vi "LcError_SetError.vi"(1 "status":bool=TRUE, 2 "code (5000)":i32=5000, 3 "source":string, 5 "error in (no error)":errorcluster, 6 "UserDefinedCodes(+5000)":variant, 7 "Error SubVI Level(1)":i32=1, 8 "StartErrorCode(5000)":i32=5000) -> (19 "error out":errorcluster)   [LabVIEW 2019]
doc: "You can use this VI to generate errors.\nThe path to the calling Vi will be added in the source.\nIf you wrap this VI inside another SetError VI (E.g. MyApplication_SetError), you can change set the <B>Error SubVI Level(1)</B> to 2"
panel:
  # "If you wrap this VI inside another SetError VI (E.g. MyApplication_SetError), you can change set the <B>Error SubVI Level(1)</B> to 2"
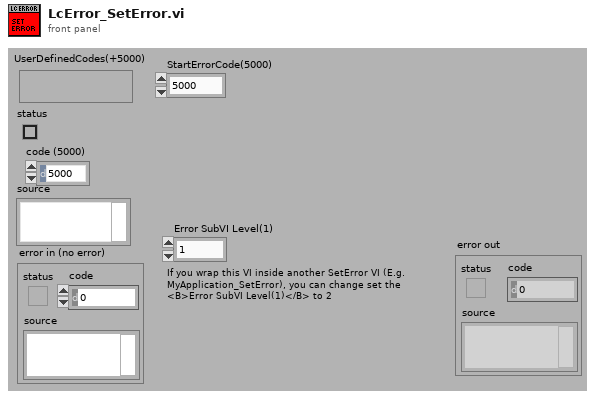
[diagram p1: front panel]
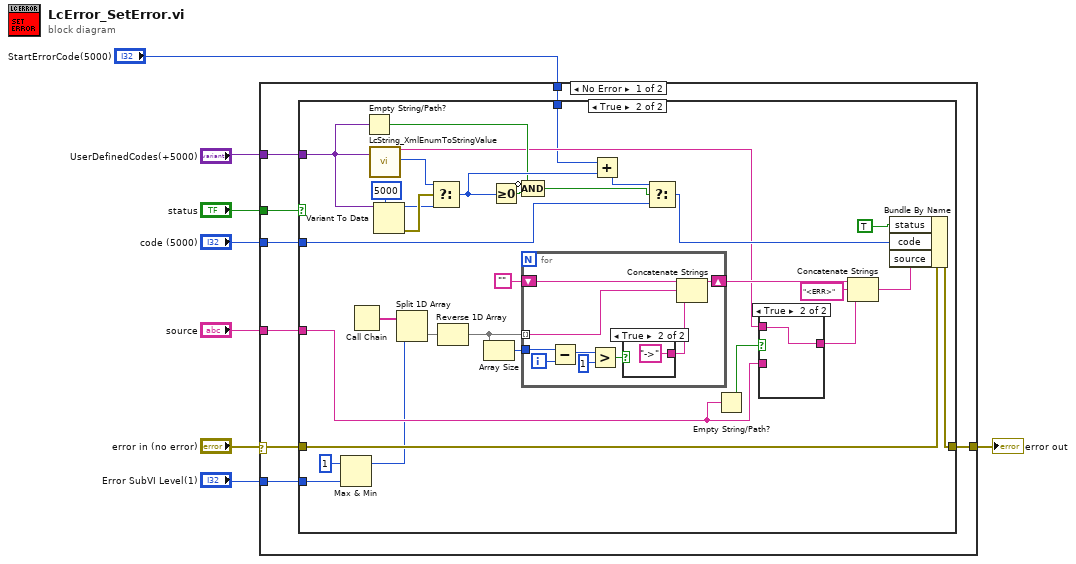
[diagram p0: block diagram]
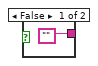
[diagram p4: hidden frame]
diagram:
  n1 = case shown="No Error" "error in (no error)" {
    selector: "error in (no error)" -> [w12 w62]
    tunnel: [w16 w62] -> w8
    tunnel: "status" -> [w15 _]
    tunnel: "code (5000)" -> [w14 _]
    tunnel: "source" -> [w13 _]
    tunnel: "UserDefinedCodes(+5000)" -> [w11 _]
    tunnel: "StartErrorCode(5000)" -> [w10 _]
    tunnel: "Error SubVI Level(1)" -> [w9 _]
    frame No Error {
      n2 = case shown="True" w15 {
        tunnel: w12 -> [w17 w48]
        tunnel: [w17 w47] -> w16
        tunnel: w14 -> [_ w36]
        tunnel: w13 -> [_ w22]
        tunnel: w11 -> [_ w26]
        tunnel: w10 -> [_ w21]
        tunnel: w9 -> [_ w19]
        frame False {
        }
        frame True {
          n3 = Max & Min(x=1, y=w19) -> (max(x,y)=w18:i32)  [unwired: 1 out]
          n4 = Call Chain() -> (call chain=w45:string[])
          n5 = Empty String/Path?(string/path=w26) -> (empty?=w27:bool)
          n6 = call "LcString_XmlEnumToStringValue.vi"("EnumVariantIn(used if String is Empty)"=w26) -> ("EnumValueOut(string)"=w24:string, "EnumValueOut(uint16)"=w30:u16)  [unwired: 2 in, 15 out]
          n7 = Variant To Data(type=5000 ("code (5000)"), Variant=w26) -> (data=w31:i32, error out=w32:errorcluster)  [unwired: 1 in]
          n8 = Split 1D Array(array=w45, index=w18) -> (second subarray=w44:string[])  [unwired: 1 out]
          n9 = Select(t=w30, s=w32, f=w31) -> (s? t:f=w29:i32)
          n10 = Reverse 1D Array(array=w44) -> (reversed array=w38:string[])
          n11 = Array Size(array=w38) -> (size(s)=w43:i32)
          n12 = Greater Or Equal To 0?(x=w29) -> (x >= 0?=w37:bool)
          n13 = Compound Arithmetic op=AND(invert w27, w37) -> (w28:bool)
          n14 = for {
            shift-right: [w51] -> w41
            shift-left: "" -> [w54]
            tunnel: w38 -> [w52] mode=indexing
            tunnel: w43 -> [w59]
            i -> [w58]
            n15 = Subtract(x=w59, y=w58) -> (x-y=w57:i32)
            n16 = Greater?(x=w57, y=1) -> (0:w55:bool)
            n17 = case shown="True" w55 {
              tunnel: ["" "->"] -> w53
              frame False {
              }
              frame True {
              }
            }
            n18 = Concatenate Strings(w54, w52, w53) -> (w51:string)
          }
          n19 = Add(x=w21, y=w29) -> (x+y=w34:i32)
          n20 = Select(t=w34, s=w28, f=w36) -> (s? t:f=w35:i32)
          n21 = Empty String/Path?(string/path=w22) -> (empty?=w25:bool)
          n22 = case shown="True" w25 {
            tunnel: w24 -> [_ w50]
            tunnel: w22 -> [w49 _]
            tunnel: [w49 w50] -> w23
            frame False {
            }
            frame True {
            }
          }
          n23 = Concatenate Strings(w41, "<ERR>" ("Substring"), w23) -> (w42:string)
          n24 = Bundle By Name(cluster=w48, "status"=TRUE ("Bundle Element"), "code"=w35, "source"=w42) -> (w47:errorcluster)
        }
      }
    }
    frame Error {
    }
  }
  "error out" <- w8
